vi "LocationDialog.vi"(10 "Info":cluster{"Set":string, "Position":i32, "Tap":i32}) -> (1 "Pause?":bool, 2 "Redo?":bool)   [LabVIEW 2022 SP3]
panel:
  in  "Pause":bool
  out "Text":string
  in  "Next Location":bool
  in  "Redo":bool
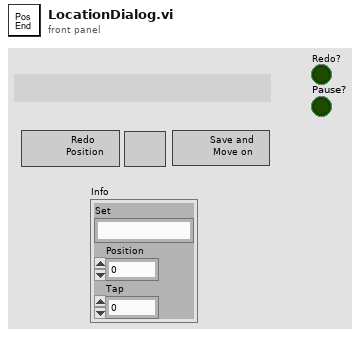
[diagram p1: front panel]
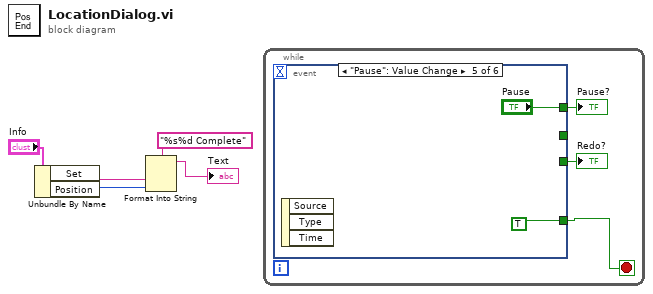
[diagram p0: block diagram]
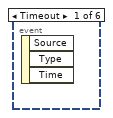
[diagram p2: hidden frame]
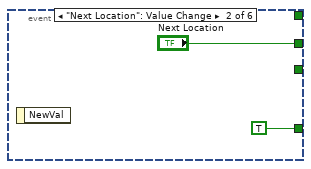
[diagram p3: hidden frame]
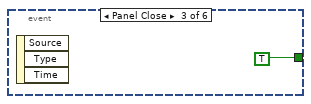
[diagram p4: hidden frame]
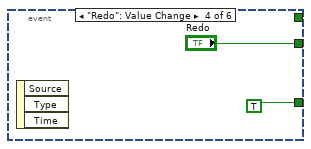
[diagram p5: hidden frame]
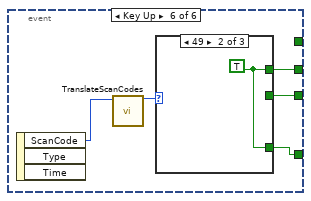
[diagram p6: hidden frame]
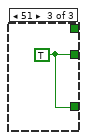
[diagram p8: hidden frame]
diagram:
  n1 = Unbundle By Name("Info") -> ("Set"=w4:string, "Position"=w5:i32)
  n2 = Format Into String(format string="%s%d Complete" ("Text"), w4, w5) -> (resulting string=→"Text":string)  [unwired: 2 in, 1 out]
  n3 = while {
    stop <- w7 stop-if-true
    n4 = event shown="[4] \"Pause\": Value Change" {
      selector: _ -> [_ _ _ _ _ _]
      dyn-events: _ -> [_ _ _ _ _ _]
      timeout: _ -> [_ _ _ _ _ _]
      tunnel: [_ "Next Location" _ _ _ w20] -> _
      tunnel: [_ _ _ "Redo" _ w19] -> w8
      tunnel: [_ TRUE ("Redo") TRUE ("Redo") TRUE ("Redo") TRUE ("Redo") w16] -> w7
      tunnel: [_ _ _ _ "Pause" _] -> w6
      event Timeout {
        n5 = event-data() -> ()  [unwired: 1 in, 3 out]
      }
      event "Next Location": Value Change {
        n6 = event-data() -> ()  [unwired: 1 in, 1 out]
      }
      event Panel Close {
        n7 = event-data() -> ()  [unwired: 1 in, 3 out]
      }
      event "Redo": Value Change {
        n8 = event-data() -> ()  [unwired: 1 in, 3 out]
      }
      event "Pause": Value Change {
        n9 = event-data() -> ()  [unwired: 1 in, 3 out]
      }
      event Key Up {
        n10 = event-data() -> ("ScanCode"=w18:i16)  [unwired: 1 in, 2 out]
        n11 = call "TranslateScanCodes.vi"("ScanCode in"=w18) -> ("ScanCode out"=w17:i16)  [unwired: 10 in]
        n12 = case shown="49" w17 {
          tunnel: [_ w21 _] -> w20
          tunnel: [_ _ w22] -> w19
          tunnel: [_ w21 w22] -> w16
          frame 0, Default {
          }
          frame 49 {
            w21 = TRUE
          }
          frame 51 {
            w22 = TRUE
          }
        }
      }
    }
    "Redo?" <- w8
    "Pause?" <- w6
  }
